vi "get_charge.vi"(11 "Data In":string) -> (3 "Data Out":string)   [LabVIEW 2018, in "Labview Python.lvlib"]
uses:
  Labview Python.lvlib
  Mass Analysis/Mass Analysis.lvlib
panel:
  out "JSON string":string
  out "Frequency vs Scan":T1(graph)
  out "Certainty of First Q State":T2(graph)
  in  "output cluster 2":T3
  in  "output cluster":T4
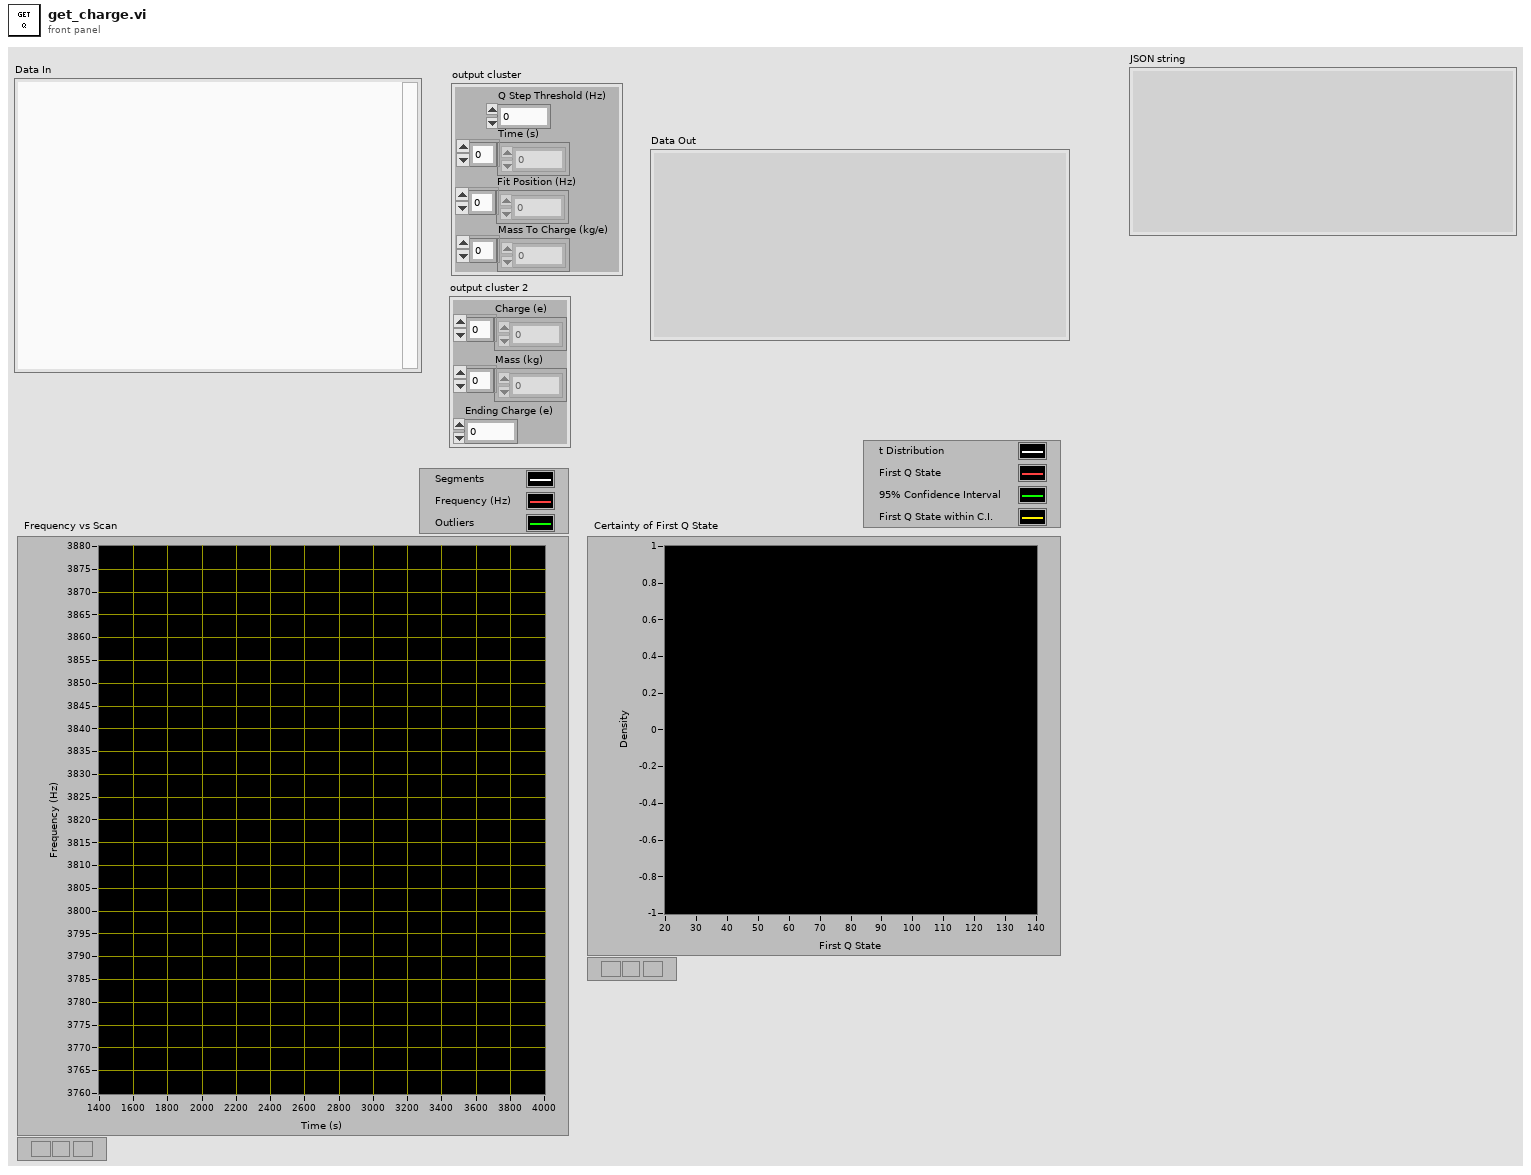
[diagram p1: front panel]
types:
  T1 = cluster{"Scan #":dbl[], "Fit Position (Hz)":dbl[]}[]
  T2 = cluster{"Ramp Pattern":dbl[], "All First Q States":dbl[]}[]
  T3 = cluster{"Charge (e)":dbl[], "Mass (kg)":dbl[], "Ending Charge (e)":dbl}
  T4 = cluster{"Q Step Threshold (Hz)":dbl, "Time (s)":dbl[], "Fit Position (Hz)":dbl[], "Mass To Charge (kg/e)":dbl[]}
  T5 = cluster{"Mean First Q State":dbl, "Mean Step Size":dbl, "Standard Error Step Size":dbl, "Standard Error Q State":dbl, "All First Q State":dbl[]}
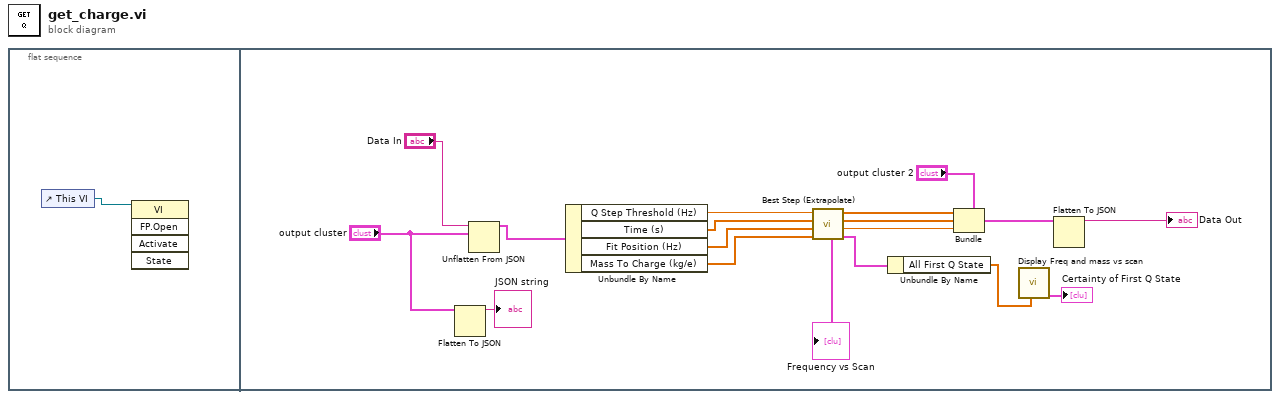
[diagram p0: block diagram]
diagram:
  n1 = flat-sequence {
    frame #0 {
      n2 = control-ref of="This VI"() -> (w1:refnum<vi>)
      n3 = invoke class="VI" method="FP.Open"(reference=w1) -> ()  [unwired: 4 in, 5 out]
    }
    frame #1 {
      n4 = Flatten To JSON(anything="output cluster") -> (JSON string=→"JSON string":string)  [unwired: 2 in, 1 out]
      n5 = Unflatten From JSON(JSON string="Data In", type and defaults="output cluster") -> (value=w18:T4)  [unwired: 5 in, 1 out]
      n6 = Unbundle By Name(w18) -> ("Q Step Threshold (Hz)"=w17:dbl, "Time (s)"=w11:dbl[], "Fit Position (Hz)"=w10:dbl[], "Mass To Charge (kg/e)"=w16:dbl[])
      n7 = call "Best Step (Extrapolate).vi"("Mass/Q (kg/e)"=w16, "Fit Position (Hz)"=w10, "Time (s)"=w11, "Q Step Threshold (Hz)"=w17) -> ("Q State Statistics Out"=w3:T5, "Ending Charge (e)"=w14:dbl, "Mass (kg) Out"=w8:dbl[], "Charge (e) Out"=w9:dbl[], "Frequency vs Scan"=→"Frequency vs Scan":T1)  [unwired: 3 in]
      n8 = Unbundle By Name(w3) -> ("All First Q State"=w2:dbl[])
      n9 = Bundle(cluster="output cluster 2", "Charge (e)"=w9, "Mass (kg)"=w8, "Ending Charge (e)"=w14) -> (w12:T3)
      n10 = call "Display Freq and mass vs scan.vi"("Charge steps.All First Q States"=w2) -> ("Certainty of First Q State"=→"Certainty of First Q State":T2)  [unwired: 7 in, 3 out]
      n11 = Flatten To JSON(anything=w12) -> (JSON string=→"Data Out":string)  [unwired: 2 in, 1 out]
    }
  }
